vi "dataProcessing.vi"(2 "中频信号":dbl[](array[numeric]), 3 "参考信号":dbl[](array[numeric])) -> (0 "mean_Q":dbl, 1 "mean_I":dbl)   [LabVIEW 2018]
uses:
  <vilib>/Analysis/3filter.llb/FIR Filter (DBL).vi
  <vilib>/Analysis/NI_AALPro.lvlib
  <vilib>/Analysis/NI_AALBase.lvlib
panel:
  in  "输入数组":dbl[](array[numeric])=[0.00773694390696, 0.0101473954367195, 0.0171175402006959, 0.0278920548608352, 0.041303353569927, 0.055898114015113, 0.0700947674411091, 0.0823548861654153, 0.0913498960888874, 0.0961050483143375, 0.0961050483143375, 0.0913498960888874, 0.0823548861654153, 0.0700947674411091, 0.055898114015113, 0.041303353569927, 0.0278920548608352, 0.0171175402006959, 0.0101473954367195, 0.00773694390696] format="%#_15g"
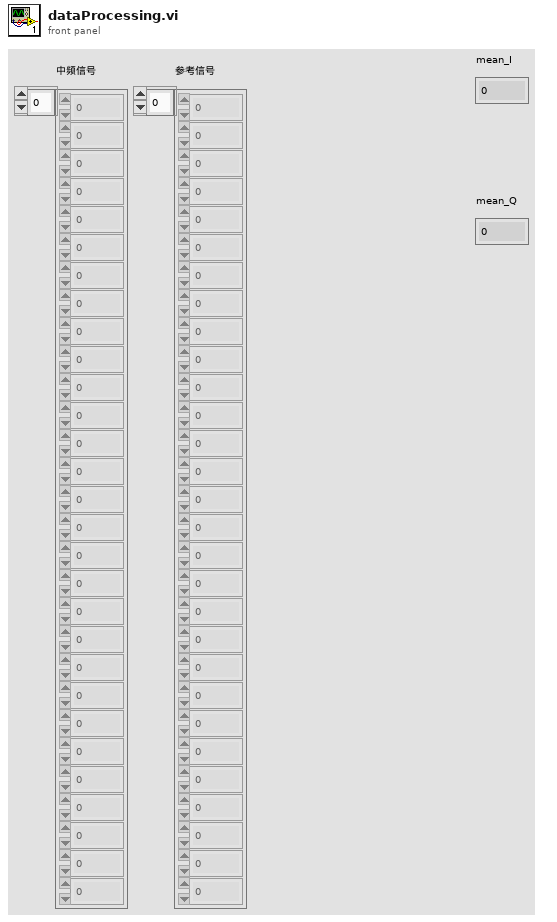
[diagram p1: front panel]
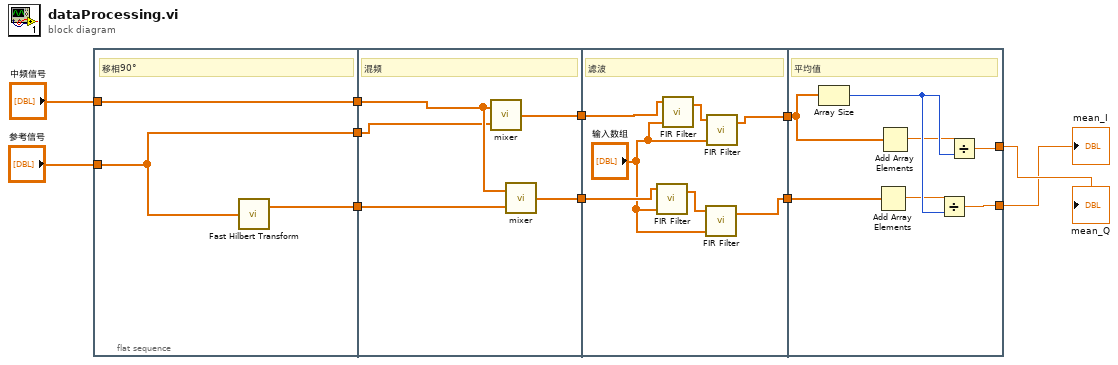
[diagram p0: block diagram]
diagram:
  n1 = flat-sequence {
    tunnel: [w13] -> w11
    tunnel: "中频信号" -> [w13]
    tunnel: "参考信号" -> [w12]
    tunnel: [w14] -> w8
    tunnel: [w12] -> w7
    tunnel: w11 -> [w19]
    tunnel: [w16] -> w10
    tunnel: [w15] -> w9
    tunnel: w8 -> [w17]
    tunnel: w7 -> [w18]
    tunnel: w10 -> [w26]
    tunnel: w9 -> [w25]
    tunnel: [w20] -> w6
    tunnel: [w21] -> w5
    tunnel: w6 -> [w31]
    tunnel: w5 -> [w29]
    tunnel: [w27] -> _
    tunnel: [w32] -> w2
    tunnel: [w27] -> w1
    frame #0 {
      # "移相90°"
      n2 = call <vilib>:"Fast Hilbert Transform.vi"("X"=w12) -> ("Hilbert{X}"=w14:dbl[])  [unwired: 1 out]
    }
    frame #1 {
      # "混频"
      n3 = call "mixer.vi"("参考信号"=w18, "中频信号"=w19) -> ("混频信号输出"=w16:dbl[])
      n4 = call "mixer.vi"("参考信号"=w17, "中频信号"=w19) -> ("混频信号输出"=w15:dbl[])
    }
    frame #2 {
      # "滤波"
      n5 = call-poly <vilib>:"FIR Filter.vi"("FIR Coefficients"="输入数组", "X"=w25) -> ("Filtered X"=w23:dbl[])  [unwired: 2 in, 1 out]
      n6 = call-poly <vilib>:"FIR Filter.vi"("FIR Coefficients"="输入数组", "X"=w26) -> ("Filtered X"=w24:dbl[])  [unwired: 2 in, 1 out]
      n7 = call-poly <vilib>:"FIR Filter.vi"("FIR Coefficients"="输入数组", "X"=w23) -> ("Filtered X"=w21:dbl[])  [unwired: 2 in, 1 out]
      n8 = call-poly <vilib>:"FIR Filter.vi"("FIR Coefficients"="输入数组", "X"=w24) -> ("Filtered X"=w20:dbl[])  [unwired: 2 in, 1 out]
    }
    frame #3 {
      # "平均值"
      n9 = Array Size(array=w31) -> (size(s)=w33:i32)
      n10 = Add Array Elements(numeric array=w29) -> (sum=w28:dbl)
      n11 = Add Array Elements(numeric array=w31) -> (sum=w30:dbl)
      n12 = Divide(x=w28, y=w33) -> (x/y=w27:dbl)
      n13 = Divide(x=w30, y=w33) -> (x/y=w32:dbl)
    }
  }
  "mean_Q" <- w2
  "mean_I" <- w1
